vi "LK340configSettle.vi"(8 "error in (no error)":errorcluster, 9 "Reading must\nStay in Band (0s)":dbl min=0.0 max=86400.0 step=1.0, 10 "Threshold (0.0000)":dbl min=0.0 max=100.0 step=0.0001 format="%.4f", 11 "VISA resource name":refnum<visa-resource-name>) -> (0 "error out":errorcluster, 3 "VISA resource name out":refnum<visa-resource-name>)   [LabVIEW 2015]
panel:
  # "Loop 1 Settle Parameters"
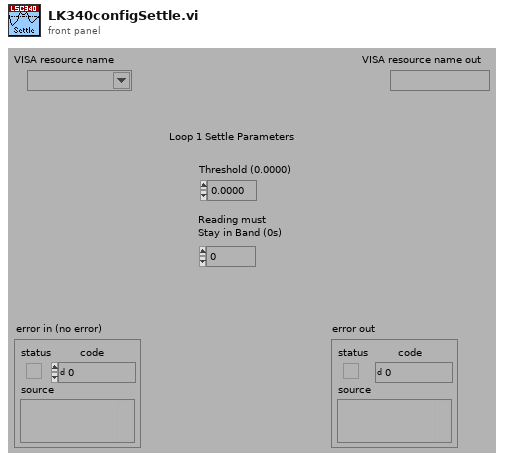
[diagram p1: front panel]
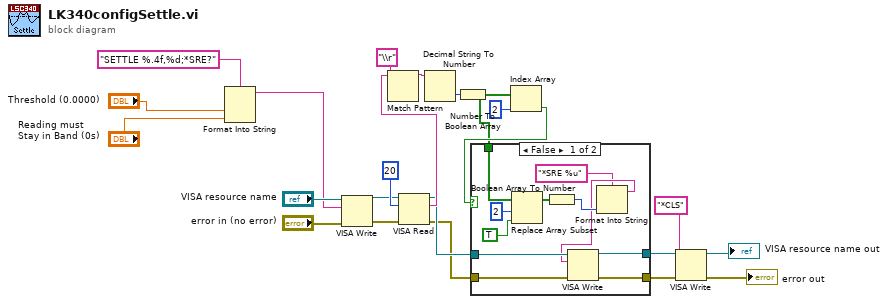
[diagram p0: block diagram]
diagram:
  n1 = Format Into String(format string="SETTLE %.4f,%d;*SRE?", "Threshold (0.0000)", "Reading must\nStay in Band (0s)") -> (resulting string=w18:string)  [unwired: 2 in, 1 out]
  n2 = VISA Write(VISA resource name="VISA resource name", write buffer=w18, error in (no error)="error in (no error)") -> (VISA resource name out=w16:refnum<visa-resource-name>, error out=w15:errorcluster)  [unwired: 1 out]
  n3 = VISA Read(VISA resource name=w16, byte count=20, error in (no error)=w15) -> (VISA resource name out=w8:refnum<visa-resource-name>, read buffer=w10:string, error out=w7:errorcluster)  [unwired: 1 out]
  n4 = Match Pattern(string=w10, regular expression="\\r") -> (before substring=w13:string)  [unwired: 4 out]
  n5 = Decimal String To Number(string=w13) -> (number=w12:i32)  [unwired: 3 out]
  n6 = Number To Boolean Array(number=w12) -> (Boolean array=w6:bool[])
  n7 = Index Array(array=w6, index=2) -> (element=w9:bool)
  n8 = case shown="False" w9 {
    tunnel: w8 -> [w29 w36]
    tunnel: [w28 w36] -> w5
    tunnel: w7 -> [w26 w35]
    tunnel: [w27 w35] -> w2
    tunnel: w6 -> [w34 _]
    frame False {
      n9 = Replace Array Subset(array=w34, new element=TRUE ("new element/subarray"), index=2) -> (w31:bool[])
      n10 = Boolean Array To Number(Boolean array=w31) -> (number=w30:u32)
      n11 = Format Into String(format string="*SRE %u", w30) -> (resulting string=w25:string)  [unwired: 2 in, 1 out]
      n12 = VISA Write(VISA resource name=w29, write buffer=w25, error in (no error)=w26) -> (VISA resource name out=w28:refnum<visa-resource-name>, error out=w27:errorcluster)  [unwired: 1 out]
    }
    frame True {
    }
  }
  n13 = VISA Write(VISA resource name=w5, write buffer="*CLS", error in (no error)=w2) -> (VISA resource name out=→"VISA resource name out":refnum<visa-resource-name>, error out=→"error out":errorcluster)  [unwired: 1 out]
